vi "BuildTileCode.vi"(4 "replacecolor 2":fxp<+,3,3>, 5 "replacecolor":fxp<+,3,3>, 6 "color_to_replace 2":fxp<+,3,3>, 7 "color_to_replace":fxp<+,3,3>, 9 "Flip":enum16{"None", "LeftRight", "UpDown", "Both"}(ring), 10 "Rotation":enum16{"None", "Right", "Down", "Left"}(ring), 11 "Tilenumber":u16) -> (3 "Tilecode":u32)   [LabVIEW 2019, in "Initializers.lvlib"]
uses:
  Initializers.lvlib
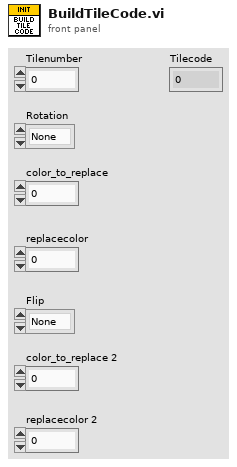
[diagram p1: front panel]
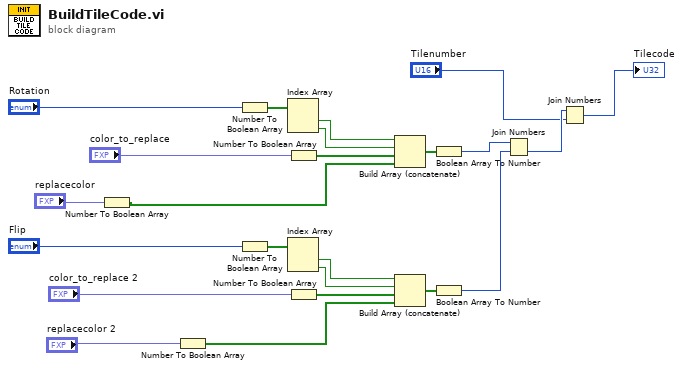
[diagram p0: block diagram]
diagram:
  n1 = Number To Boolean Array(number="replacecolor") -> (Boolean array=w3:bool[])
  n2 = Number To Boolean Array(number="replacecolor 2") -> (Boolean array=w1:bool[])
  n3 = Number To Boolean Array(number="Rotation") -> (Boolean array=w6:bool[])
  n4 = Number To Boolean Array(number="Flip") -> (Boolean array=w18:bool[])
  n5 = Index Array(array=w6) -> (element #1=w7:bool, element #2=w8:bool)  [unwired: 2 in]
  n6 = Index Array(array=w18) -> (element #1=w17:bool, element #2=w16:bool)  [unwired: 2 in]
  n7 = Number To Boolean Array(number="color_to_replace") -> (Boolean array=w9:bool[])
  n8 = Number To Boolean Array(number="color_to_replace 2") -> (Boolean array=w15:bool[])
  n9 = Build Array (concatenate)(w7, w8, w9, w3) -> (w10:bool[])
  n10 = Build Array (concatenate)(w17, w16, w15, w1) -> (w20:bool[])
  n11 = Boolean Array To Number(Boolean array=w10) -> (number=w22:u8)
  n12 = Boolean Array To Number(Boolean array=w20) -> (number=w23:u8)
  n13 = Join Numbers(hi=w22, lo=w23) -> ((hi.lo)=w21:u16)
  n14 = Join Numbers(hi=w21, lo="Tilenumber") -> ((hi.lo)=→"Tilecode":u32)
